vi "保存数据到USB.vi"   [LabVIEW 2020]
uses:
  Global variable.vi
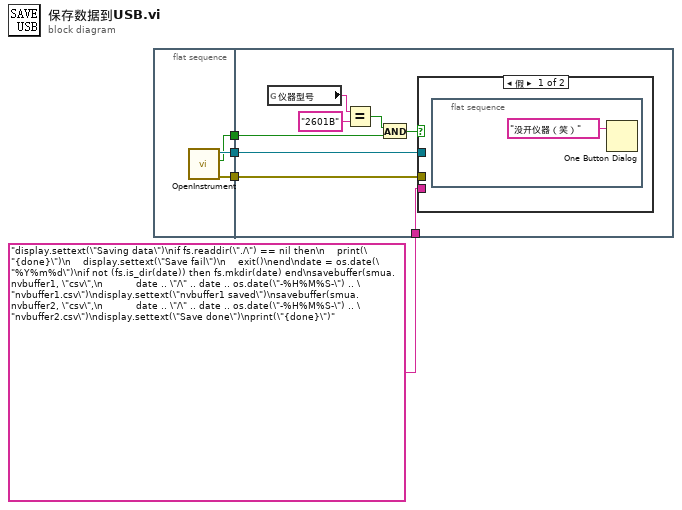
[diagram p0: block diagram]
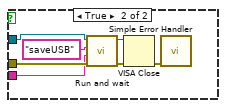
[diagram p2: hidden frame]
diagram:
  n1 = flat-sequence {
    tunnel: [w7] -> w4
    tunnel: [w6] -> w3
    tunnel: [w5] -> w2
    tunnel: w4 -> [w15]
    tunnel: w3 -> [w14]
    tunnel: w2 -> [w9]
    tunnel: "display.settext(\"Saving data\")\nif fs.readdir(\"./\") == nil then\n    print(\"{done}\")\n    display.settext(\"Save fail\")\n    exit()\nend\ndate = os.date(\"%Y%m%d\")\nif not (fs.is_dir(date)) then fs.mkdir(date) end\nsavebuffer(smua.nvbuffer1, \"csv\",\n           date .. \"/\" .. date .. os.date(\"-%H%M%S-\") .. \"nvbuffer1.csv\")\ndisplay.settext(\"nvbuffer1 saved\")\nsavebuffer(smua.nvbuffer2, \"csv\",\n           date .. \"/\" .. date .. os.date(\"-%H%M%S-\") .. \"nvbuffer2.csv\")\ndisplay.settext(\"Save done\")\nprint(\"{done}\")" ("Script") -> [w13]
    frame #0 {
      n2 = call "OpenInstrument.vi"() -> ("错误输出"=w6:errorcluster, "仪器存在"=w5:bool, "VISA资源名称输出"=w7:refnum<visa-resource-name>)  [unwired: 9 in]
    }
    frame #1 {
      n3 = global read "Global variable.vi" "仪器型号"() -> (w12:string)
      n4 = Equal?(x=w12, y="2601B") -> (x = y?=w10:bool)
      n5 = And(x=w10, y=w9) -> (x .and. y?=w8:bool)
      n6 = case shown="假" w8 {
        tunnel: w15 -> [_ w22]
        tunnel: w14 -> [_ w21]
        tunnel: w13 -> [_ w20]
        frame False {
          n7 = flat-sequence {
            frame #0 {
              n8 = One Button Dialog(message="没开仪器（笑）" ("消息")) -> ()  [unwired: 1 in, 1 out]
            }
          }
        }
        frame True {
          n9 = call "Run and wait.vi"("错误输入"=w21, "Script"=w20, "Script Name"="saveUSB", "VISA资源名称"=w22) -> ("错误输出"=w17:errorcluster, "VISA资源名称输出"=w18:refnum<visa-resource-name>)  [unwired: 6 in]
          n10 = VISA Close(VISA resource name=w18, error in (no error)=w17) -> (error out=w19:errorcluster)
          n11 = call <vilib>:"Simple Error Handler.vi"("error in (no error)"=w19) -> ()  [unwired: 4 in, 5 out]
        }
      }
    }
  }
